vi "extract_image_and_count_electrons.vi"(0 "Image Q In":T1, 11 "Electron Count Q In":T1, 12 "Range":cluster{"Lower value":sgl, "Upper value":sgl}={"Lower value"=128.0, "Upper value"=255.0} {"Upper value" format="%.2f"; "Lower value" format="%.2f"}) -> (4 "Image Q Out":T1, 14 "error out":errorcluster, 15 "Electron Count Q Out":T1)   [LabVIEW 2023]
uses:
  <vilib>/vision/Image Controls.llb/IMAQ Image.ctl
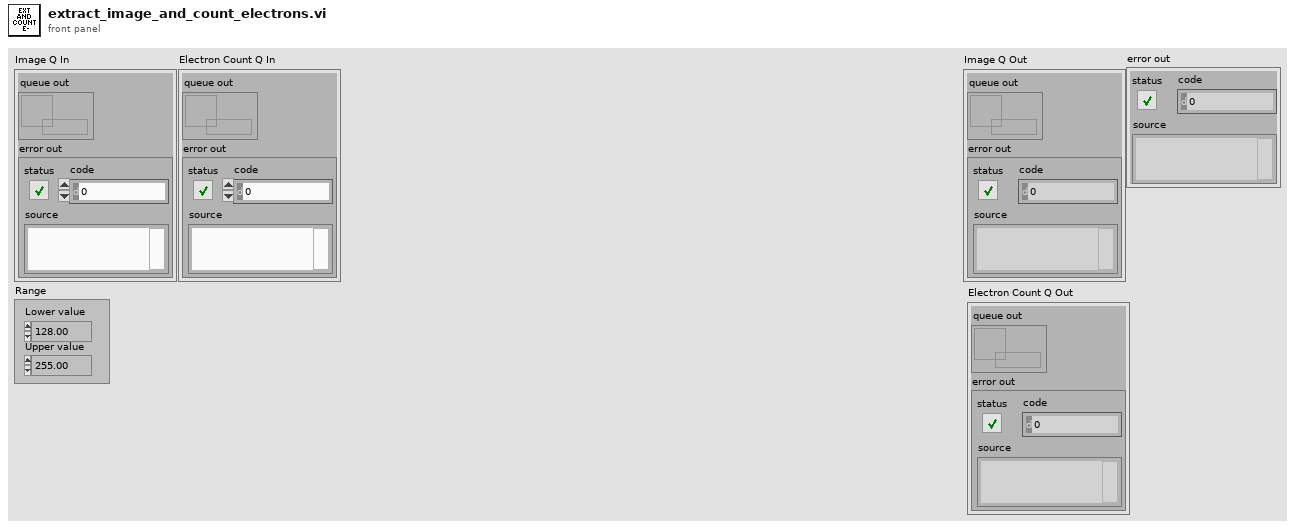
[diagram p1: front panel]
types:
  T1 = cluster{"queue out":refnum<queue>, "error out":errorcluster}
  T2 = typedef "IMAQ Image.ctl" = refnum<image>
  T3 = cluster{"Image Out":T2, "Image Data":cluster{"Actual Width":u32, "Actual Height":u32, "Buffer Number":i32}, "Imaging Variables In":cluster{"Region of interest":i32[], "Number of buffers":u32, "Frame timeout (ms)":u32}}
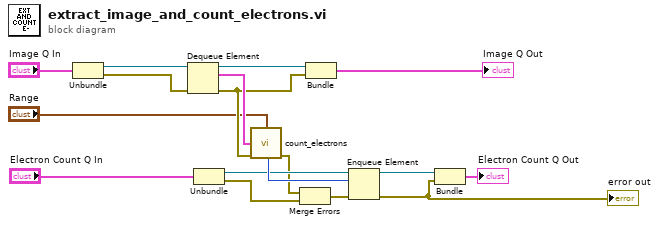
[diagram p0: block diagram]
diagram:
  n1 = Unbundle("Image Q In") -> ("queue out"=w16:refnum<queue>, "error out"=w15:errorcluster)
  n2 = Dequeue Element(queue=w16, error in (no error)=w15) -> (queue out=w14:refnum<queue>, element=w12:T3, error out=w3:errorcluster)  [unwired: 1 in, 1 out]
  n3 = Unbundle("Electron Count Q In") -> ("queue out"=w9:refnum<queue>, "error out"=w4:errorcluster)
  n4 = call "count_electrons.vi"("Range"="Range", "Raw Image Data In"=w12, "error in (no error)"=w3) -> ("Electron Counts Out"=w11:i32, "error out"=w2:errorcluster)  [unwired: 10 in, 1 out]
  n5 = Merge Errors(w2, w4) -> (w5:errorcluster)
  n6 = Bundle("queue out"=w14, "error out"=w3) -> (→"Image Q Out":T1)  [unwired: 1 in]
  n7 = Enqueue Element(queue=w9, element=w11, error in (no error)=w5) -> (queue out=w8:refnum<queue>, error out=w7:errorcluster)  [unwired: 1 in, 1 out]
  "error out" <- w7
  n8 = Bundle("queue out"=w8, "error out"=w7) -> (→"Electron Count Q Out":T1)  [unwired: 1 in]
